vi "CheckForErrors.vi"() -> (2 "Symbols":i32[](array[numeric]), 3 "Logs":string[][](array[string]), 4 "Paths":path[](array[path]))   [LabVIEW 2012]
doc: "Checks logs for errors"
panel:
  in  "Options":i32(listbox)
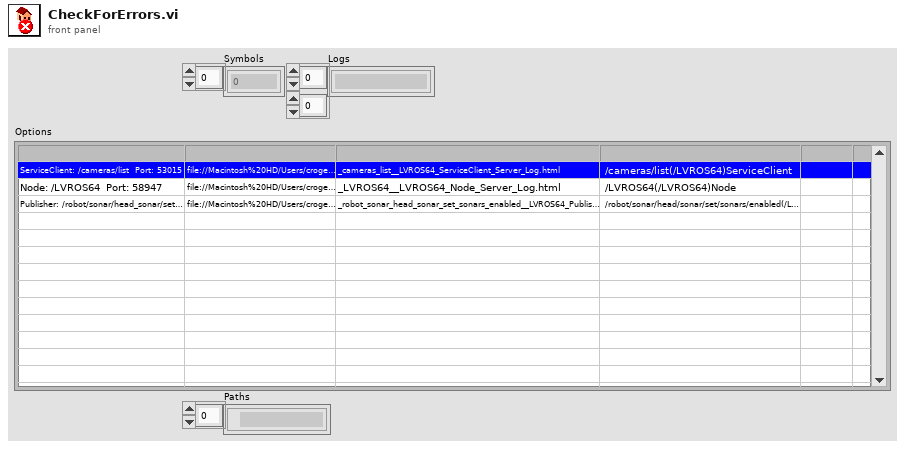
[diagram p1: front panel]
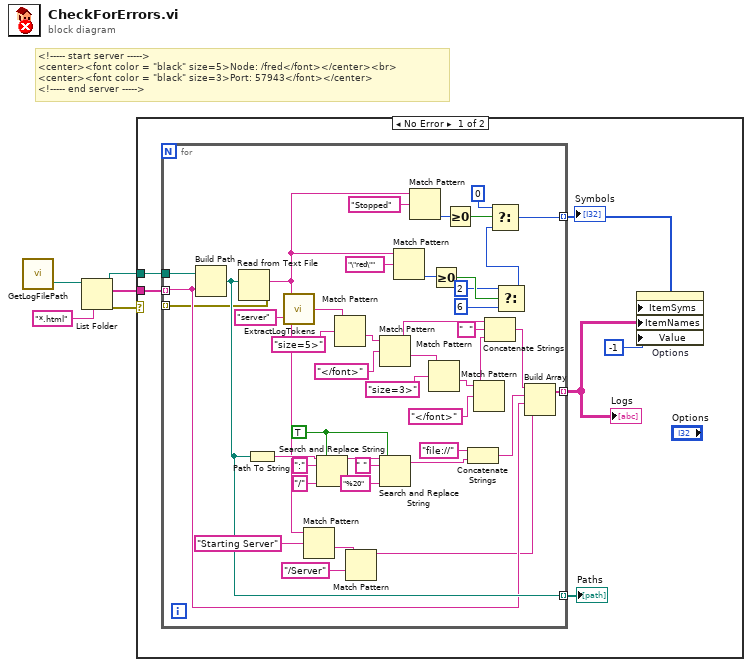
[diagram p0: block diagram]
diagram:
  # "<!----- start server ----->\n<center><font color = \"black\" size=5>Node: /fred</font></center><br>\n<center><font color = \"black\" size=3>Port: 57943</font></center> \n<!----- end server ----->"
  n1 = call <userlib>:"GetLogFilePath.vi"() -> ("LogFolder"=w5:path)  [unwired: 2 in, 1 out]
  n2 = List Folder(path=w5, pattern="*.html") -> (path out=w2:path, filenames=w3:string[], error out=w1:errorcluster)  [unwired: 2 in, 1 out]
  n3 = case shown="No Error" w1 {
    tunnel: w3 -> [w11 _]
    tunnel: w2 -> [w10 _]
    frame No Error {
      n4 = for {
        tunnel: w11 -> [w18] mode=indexing
        tunnel: w10 -> [w44]
        tunnel: [w20] -> w9 mode=indexing
        tunnel: [w26] -> w7 mode=indexing
        tunnel: [w19] -> w6 mode=indexing
        tunnel: [w17] -> _ mode=indexing
        w36 = TRUE ("replace all? (F)")
        n5 = Build Path(base path=w44, name or relative path=w18) -> (appended path=w19:path)
        n6 = Read from Text File(file (use dialog)=w19) -> (text=w16:string, error out=w17:errorcluster)  [unwired: 3 in, 2 out]
        n7 = Path To String(path=w19) -> (string=w30:string)
        n8 = call <userlib>:"ExtractLogTokens.vi"("HTML"=w16, "section"="server" ("string")) -> ("tagged text"=w54:string)  [unwired: 2 out]
        n9 = Match Pattern(string=w16, regular expression="Starting Server") -> (after substring=w15:string)  [unwired: 1 in, 3 out]
        n10 = Search and Replace String(replace all?=w36, input string=w30, search string=":", replace string="/" ("replace string (\"\")")) -> (result string=w35:string)  [unwired: 4 in, 3 out]
        n11 = Match Pattern(string=w54, regular expression="size=5>") -> (after substring=w52:string)  [unwired: 1 in, 3 out]
        n12 = Match Pattern(string=w15, regular expression="/Server") -> (before substring=w13:string)  [unwired: 1 in, 3 out]
        n13 = Match Pattern(string=w52, regular expression="</font>") -> (before substring=w46:string, after substring=w47:string)  [unwired: 1 in, 2 out]
        n14 = Search and Replace String(replace all?=w36, input string=w35, search string=" ", replace string="%20" ("replace string (\"\")")) -> (result string=w37:string)  [unwired: 4 in, 3 out]
        n15 = Match Pattern(string=w16, regular expression="\"red\"") -> (offset past match=w41:i32)  [unwired: 1 in, 3 out]
        n16 = Match Pattern(string=w16, regular expression="Stopped") -> (offset past match=w24:i32)  [unwired: 1 in, 3 out]
        n17 = Match Pattern(string=w47, regular expression="size=3>") -> (after substring=w49:string)  [unwired: 1 in, 3 out]
        n18 = Greater Or Equal To 0?(x=w41) -> (x >= 0?=w40:bool)
        n19 = Greater Or Equal To 0?(x=w24) -> (x >= 0?=w23:bool)
        n20 = Concatenate Strings("file://" ("string"), w37) -> (w27:string)
        n21 = Match Pattern(string=w49, regular expression="</font>") -> (before substring=w45:string)  [unwired: 1 in, 3 out]
        n22 = Concatenate Strings(w46, "  " ("string"), w45) -> (w28:string)
        n23 = Select(t=2, s=w40, f=6) -> (s? t:f=w21:i32)
        n24 = Select(t=0, s=w23, f=w21) -> (s? t:f=w20:i32)
        n25 = Build Array(w28, w27, w18, w13) -> (w26:string[])
      }
      "Symbols" <- w9
      "Logs" <- w7
      "Paths" <- w6
      n26 = property on="Options" class="MCListbox (strict)"("ItemSyms"=w9, "ItemNames"=w7, "Value"=-1 ("Listbox")) -> ()  [unwired: 2 in, 2 out]
    }
    frame Error {
    }
  }
